vi "7-OCU.vi"() -> ()   [LabVIEW 2010]
uses:
  4-High Neurons/4.0-Timing Badass.ctl
  7-OCU/7.0 GUI/7.0 Manual Mode Display.ctl
  6-OCU Neurons/6.1-UDP Saitek.ctl
  <vilib>/robotics/Controls/Compass Indicator/Compass Indicator.xctl
  7-OCU/7.0-OCU State.ctl
  7-OCU/7.0 GUI/7.0 Auto Mode Display.ctl
  7-OCU/7.0 GUI/7.0 Manual Mode Buttons.ctl
  7-OCU/7.0 GUI/7.0 Auto Mode Buttons.ctl
  7-OCU/7.0-Global.vi
panel:
  in  "Tab Control":T1(tab)
  out "7.0 Manual Mode GUI":T2 {"Speed (m/s)" scale=0.0..2.5; "Battery" scale=22.0..24.0; "6.1-Saitek Controller"."Right" scale=0.0..1.0; "6.1-Saitek Controller"."Left" scale=0.0..1.0; "6.1-Saitek Controller"."Yaw" scale=-1.0..1.0; "6.1-Saitek Controller"."Roll" scale=-1.0..1.0; "6.1-Saitek Controller"."Pitch" scale=-1.0..1.0}
  in  "7.0-Manual Mode Controls":T4
  out "7.0 Auto Mode Display":T5 {"Speed (m/s)" scale=0.0..2.5; "Battery" scale=20.0..24.0}
  in  "7.0 Auto Mode Controls":T6
  out "7.0 OCU State":T7
  out "GUI Heart Beat":T8
  in  "Shutdown":bool
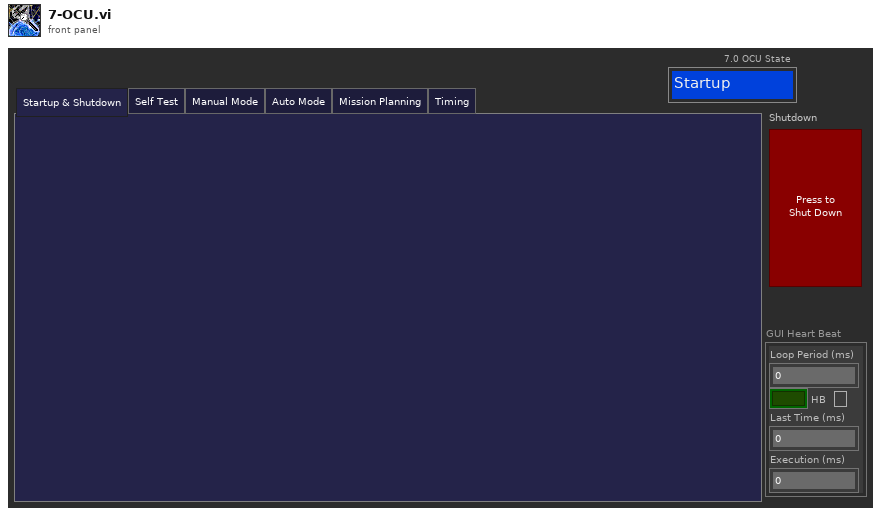
[diagram p1: front panel]
types:
  T1 = enum32{"Startup & Shutdown", "Self Test", "Manual Mode", "Auto Mode", "Mission Planning", "Timing"}
  T2 = typedef "7.0 Manual Mode Display.ctl" = cluster{"6.1-Saitek Controller":T3, "Time":dbl, "Battery":dbl, "Speed (m/s)":dbl, "Heading":dbl}
  T3 = typedef "6.1-UDP Saitek.ctl" = cluster{"Stop":bool, "Setpoint":bool, "Run":bool, "Restart":bool, "Shutdown":bool, "Joystick\nMode 1":bool, "Joystick\nMode 2":bool, "Joystick \nMode 3":bool, "Joystick Mode 4":bool, "10":bool, "11":bool, "Pitch":sgl, "Roll":sgl, "Yaw":sgl, "Left":sgl, "Right":sgl}
  T4 = typedef "7.0 Manual Mode Buttons.ctl" = cluster{"Joystick Mode":bool, "Reset":bool, "Begin":bool}
  T5 = typedef "7.0 Auto Mode Display.ctl" = cluster{"Shutdown CMD":bool, "Time":dbl, "Battery":dbl, "Speed (m/s)":dbl, "Heading":dbl, "XY Graph":cluster{dbl, dbl}[], "Latitude":dbl, "Longitude":dbl, "Lattitude of Waypoint":dbl, "Longitude of Waypoint":dbl, "Distance to Waypoint":dbl, "Has Mission Def":bool}
  T6 = typedef "7.0 Auto Mode Buttons.ctl" = cluster{"Enable Joystick":bool, "End Run":bool, "Begin":bool, "Send Map":bool}
  T7 = typedef "7.0-OCU State.ctl" = enum16{"Startup", "Self Test", "Manual Mode", "Auto Mode", "Plan Mission", "Shutdown"}
  T8 = typedef "4.0-Timing Badass.ctl" = cluster{"Loop Period (ms)":u32, "HB":bool, "Last Time (ms)":u32, "Execution (ms)":u32}
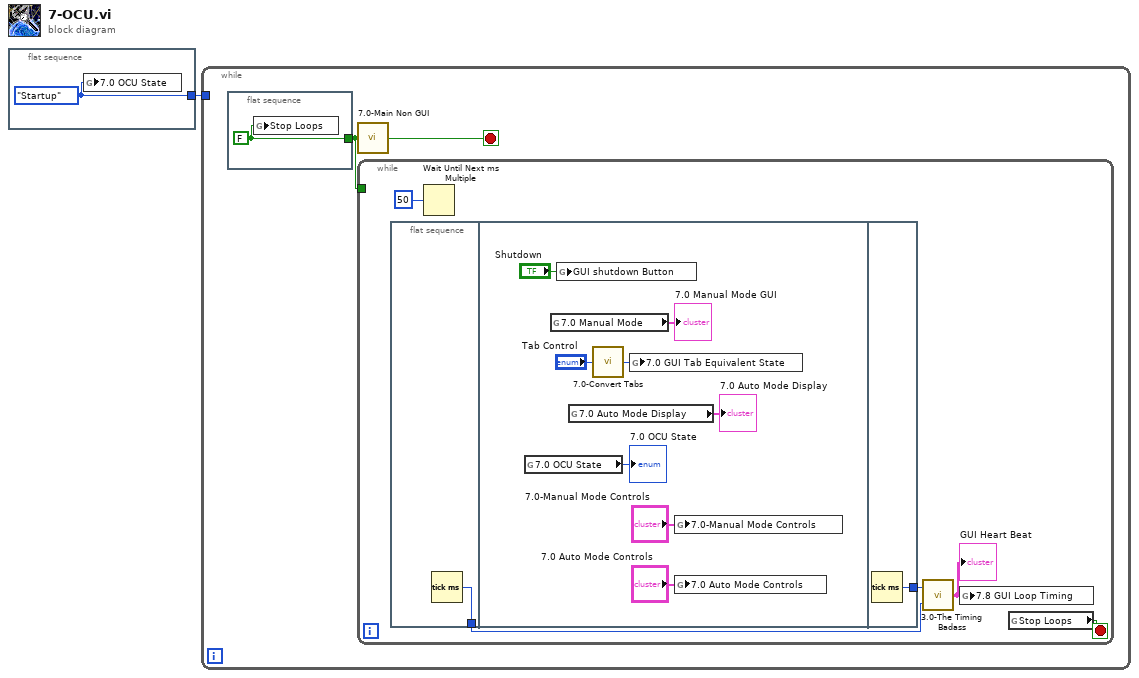
[diagram p0: block diagram]
diagram:
  n1 = flat-sequence {
    tunnel: [w2] -> w1
    frame #0 {
      w2 = 7.0-OCU_State."Startup" ("7.0 OCU State")
      n2 = global write "7.0-Global.vi" "7.0 OCU State"(w2) -> ()
    }
  }
  n3 = while {
    tunnel: w1 -> [_]
    stop <- w3 stop-if-true
    n4 = flat-sequence {
      tunnel: [w5] -> w4
      frame #0 {
        w5 = FALSE ("Stop Loops")
        n5 = global write "7.0-Global.vi" "Stop Loops"(w5) -> ()
      }
    }
    n6 = call "7.0-Main Non GUI.vi"("Begin (for Flow)"=w4) -> ("End Program"=w3:bool)
    n7 = while "7.0 GUI Loop" {
      tunnel: w4 -> [_]
      stop <- w9 stop-if-true
      n8 = flat-sequence {
        tunnel: [w11] -> w7
        tunnel: [w20] -> w8
        frame #0 {
          n9 = Tick Count (ms)() -> (millisecond timer value=w11:u32)
        }
        frame #1 {
          n10 = global read "7.0-Global.vi" "7.0 OCU State"() -> (→"7.0 OCU State":T7)
          n11 = global read "7.0-Global.vi" "7.0 Manual Mode"() -> (→"7.0 Manual Mode GUI":T2)
          n12 = global write "7.0-Global.vi" "GUI shutdown Button"("Shutdown") -> ()
          n13 = global read "7.0-Global.vi" "7.0 Auto Mode Display"() -> (→"7.0 Auto Mode Display":T5)
          n14 = call "7.0-Convert Tabs.vi"("Tab Control"="Tab Control") -> ("7.0 GUI Tab Equivalent State"=w14:T7)
          n15 = global write "7.0-Global.vi" "7.0 GUI Tab Equivalent State"(w14) -> ()
          n16 = global write "7.0-Global.vi" "7.0-Manual Mode Controls"("7.0-Manual Mode Controls") -> ()
          n17 = global write "7.0-Global.vi" "7.0 Auto Mode Controls"("7.0 Auto Mode Controls") -> ()
        }
        frame #2 {
          n18 = Tick Count (ms)() -> (millisecond timer value=w20:u32)
        }
      }
      n19 = Wait Until Next ms Multiple(millisecond multiple=u32 50) -> ()  [unwired: 1 out]
      n20 = call "3.0-The Timing Badass.vi"("Start"=w7, "End"=w8) -> ("Super Heart Beat"=w6:T8)
      "GUI Heart Beat" <- w6
      n21 = global write "7.0-Global.vi" "7.8 GUI Loop Timing"(w6) -> ()
      n22 = global read "7.0-Global.vi" "Stop Loops"() -> (w9:bool)
    }
  }
